vi "Get one point.vi"(7 "level":dbl=2.5 format="%#_13g", 8 "error in (no error)":errorcluster, 9 "Sample Rate":dbl=500000.0 format="%.3p", 10 "Voltage Read":tag="Dev1/ai1", 11 "Gate":tag="Dev1/ao0") -> (0 "error out":errorcluster, 3 "data":dbl format="%0.2f")   [LabVIEW 2017]
uses:
  <vilib>/DAQmx/read.llb/DAQmx Read (Analog DBL 1Chan 1Samp).vi
  <vilib>/DAQmx/write.llb/DAQmx Write (Analog DBL 1Chan 1Samp).vi
  <vilib>/DAQmx/create/channels.llb/DAQmx Create Channel (AI-Voltage-Basic).vi
  <vilib>/DAQmx/configure/timing.llb/DAQmx Timing (Sample Clock).vi
  <vilib>/DAQmx/configure/trigger.llb/DAQmx Start Trigger (Analog Edge).vi
  <vilib>/DAQmx/create/channels.llb/DAQmx Create Channel (AO-Voltage-Basic).vi
  <vilib>/DAQmx/configure/trigger.llb/DAQmx Start Trigger (Digital Edge).vi
  <vilib>/DAQmx/miscellaneous.llb/DAQmx Fill In Error Info.vi
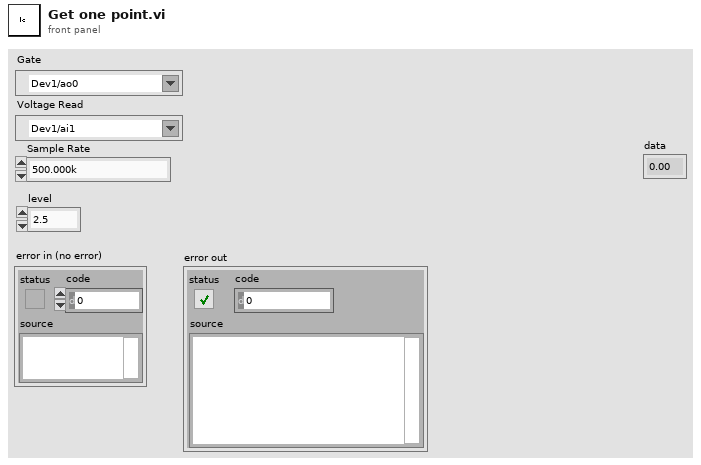
[diagram p1: front panel]
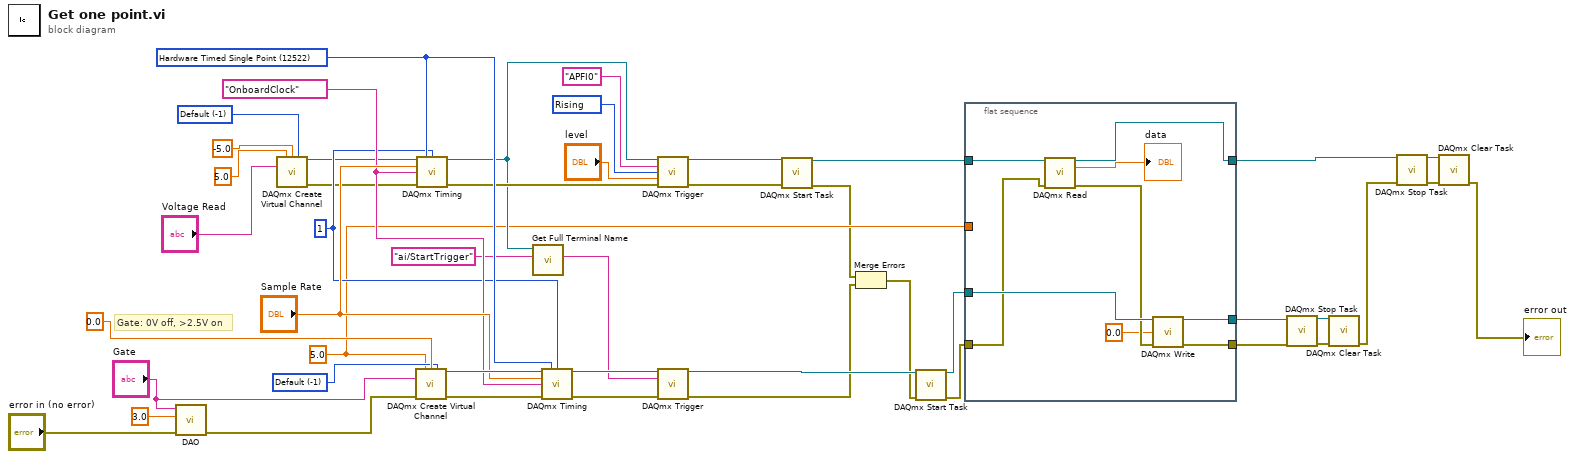
[diagram p0: block diagram]
diagram:
  w15 = 10280 items=["Rising"=10280, "Falling"=10171] ("slope")
  w33 = -1 items=["Default"=-1, "RSE"=10083, "NRSE"=10078, "Differential"=10106, "Pseudodifferential"=12529] ("input terminal configuration")
  w39 = 1 ("samples per channel")
  w40 = 12522 items=["Finite Samples"=10178, "Continuous Samples"=10123, "Hardware Timed Single Point"=12522] ("sample mode")
  w41 = tag "OnboardClock" ("source")
  w45 = -1 items=["Default"=-1, "RSE"=10083, "Differential"=10106, "Pseudodifferential"=12529] ("output terminal configuration")
  w8 = 5.0 ("maximum value")
  # "Gate: 0V off, >2.5V on"
  n1 = call "DAO.vi"("error in"="error in (no error)", "Voltage"=3.0, "Physical Channel(s)"="Gate") -> ("error out"=w12:errorcluster)  [unwired: 8 in]
  n2 = call-poly <vilib>:"DAQmx Create Virtual Channel.vi"("maximum value"=5.0, "minimum value"=-5.0, "input terminal configuration"=w33, "physical channels"="Voltage Read") -> ("task out"=w32:refnum<k21>, "error out"=w31:errorcluster)  [unwired: 10 in]
  n3 = call-poly <vilib>:"DAQmx Create Virtual Channel.vi"("maximum value"=w8, "minimum value"=0.0, "output terminal configuration"=w45, "physical channels"="Gate", "error in"=w12) -> ("task out"=w44:refnum<k21>, "error out"=w43:errorcluster)  [unwired: 9 in]
  n4 = call-poly <vilib>:"DAQmx Timing.vi"("task/channels in"=w32, "sample mode"=w40, "samples per channel"=w39, "rate"="Sample Rate", "source"=w41, "error in"=w31) -> ("task out"=w19:refnum<k21>, "error out"=w30:errorcluster)  [unwired: 8 in]
  n5 = call "Get Full Terminal Name.vi"("Local Terminal Name"="ai/StartTrigger", "task/channels in"=w19) -> ("Terminal Name with Device Prefix"=w16:tag)  [unwired: 7 in, 2 out]
  n6 = call-poly <vilib>:"DAQmx Timing.vi"("task/channels in"=w44, "sample mode"=w40, "samples per channel"=w39, "rate"="Sample Rate", "source"=w41, "error in"=w43) -> ("task out"=w38:refnum<k21>, "error out"=w37:errorcluster)  [unwired: 8 in]
  n7 = call-poly <vilib>:"DAQmx Trigger.vi"("task/channels in"=w19, "source"="APFI0", "slope"=w15, "level"="level", "error in"=w30) -> ("task out"=w29:refnum<k21>, "error out"=w28:errorcluster)  [unwired: 9 in]
  n8 = call-poly <vilib>:"DAQmx Trigger.vi"("task/channels in"=w38, "source"=w16, "error in"=w37) -> ("task out"=w21:refnum<k21>, "error out"=w3:errorcluster)  [unwired: 11 in]
  n9 = call <vilib>:"DAQmx Start Task.vi"("task/channels in"=w29, "error in"=w28) -> ("task out"=w26:refnum<k21>, "error out"=w4:errorcluster)  [unwired: 12 in]
  n10 = Merge Errors(w4, w3) -> (w2:errorcluster)
  n11 = call <vilib>:"DAQmx Start Task.vi"("task/channels in"=w21, "error in"=w2) -> ("task out"=w27:refnum<k21>, "error out"=w11:errorcluster)  [unwired: 12 in]
  n12 = flat-sequence {
    tunnel: w27 -> [w55]
    tunnel: w26 -> [w54]
    tunnel: w11 -> [w49]
    tunnel: [w51] -> w5
    tunnel: [w52] -> w7
    tunnel: w8 -> [_]
    tunnel: [w50] -> w6
    frame #0 {
      n13 = call-poly <vilib>:"DAQmx Read.vi"("task/channels in"=w54, "error in"=w49) -> ("task out"=w52:refnum<k21>, "data"=→"data":dbl, "error out"=w48:errorcluster)  [unwired: 11 in]
      n14 = call-poly <vilib>:"DAQmx Write.vi"("task/channels in"=w55, "data"=0.0, "error in"=w48) -> ("task out"=w51:refnum<k21>, "error out"=w50:errorcluster)  [unwired: 10 in, 1 out]
    }
  }
  n15 = call <vilib>:"DAQmx Stop Task.vi"("task/channels in"=w5, "error in"=w6) -> ("task out"=w25:refnum<k21>, "error out"=w24:errorcluster)  [unwired: 12 in]
  n16 = call <vilib>:"DAQmx Clear Task.vi"("task in"=w25, "error in"=w24) -> ("error out"=w1:errorcluster)  [unwired: 13 in]
  n17 = call <vilib>:"DAQmx Stop Task.vi"("task/channels in"=w7, "error in"=w1) -> ("task out"=w23:refnum<k21>, "error out"=w22:errorcluster)  [unwired: 12 in]
  n18 = call <vilib>:"DAQmx Clear Task.vi"("task in"=w23, "error in"=w22) -> ("error out"=→"error out":errorcluster)  [unwired: 13 in]
